vi "Change State To COOKING.vi"(8 "error in (no error)":errorcluster, 11 "Root Actor in":refnum<class "Root Actor.lvclass">) -> (0 "error out":errorcluster, 3 "Root Actor out":refnum<class "Root Actor.lvclass">)   [LabVIEW 2024, in "Root Actor.lvlib" / "Root Actor.lvclass"]
uses:
  Root Actor.lvclass
  Root Actor.lvclass/Root Actor.ctl
  Chef States/Chef State Messages/Go to COOKING Msg/Go to COOKING Msg.lvclass
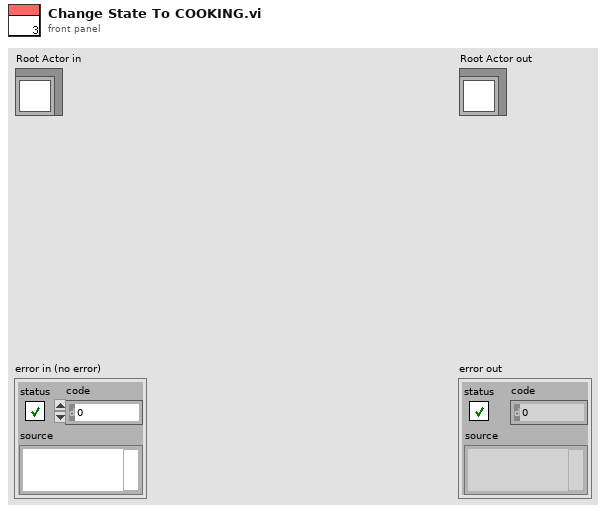
[diagram p1: front panel]
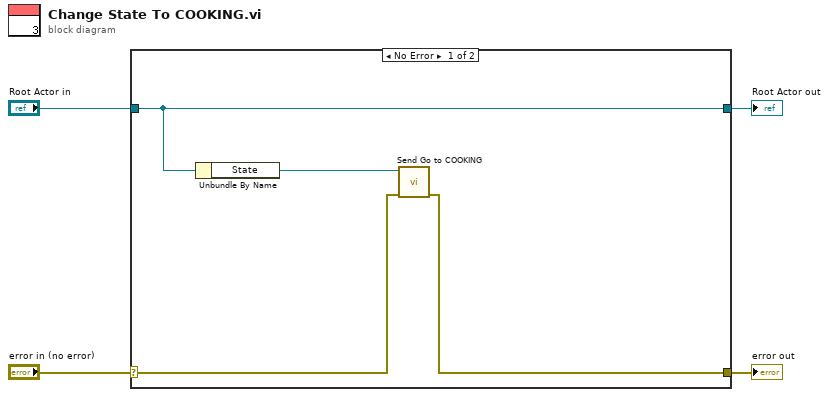
[diagram p0: block diagram]
diagram:
  n1 = case shown="No Error" "error in (no error)" {
    selector: "error in (no error)" -> [w8 w10]
    tunnel: [w6 w10] -> w3
    tunnel: [w7 w9] -> w1
    tunnel: "Root Actor in" -> [w7 w9]
    frame No Error {
      n2 = Unbundle By Name(w7) -> ("State"=w5:refnum<class "Message Enqueuer.lvclass">)
      n3 = call "Send Go to COOKING.vi"("error in (no error)"=w8, "Message Enqueuer"=w5) -> ("error out"=w6:errorcluster)  [unwired: 8 in, 1 out]
    }
    frame Error {
    }
  }
  "error out" <- w3
  "Root Actor out" <- w1
